vi "AttTGCFix.vi"(0 "slope (m)":dbl[][](array[numeric]) format="%.2f", 1 "Corrections":T1(ring), 5 "intercept (b) out":dbl[][](array[numeric]) format="%.2f", 7 "midband fit in":dbl[][](array[numeric]) format="%.2f", 9 "midband correction":dbl[](array[numeric]) format="%.2f", 11 "slope correction":dbl[](array[numeric]) format="%.2f", 13 "Fit band":T2 {"center freq" format="%.2f"; "stop freq" format="%.2f"; "start" format="%.2f"}) -> (4 "slope":dbl[][](array[numeric]) format="%.2f", 6 "intercept":dbl[][](array[numeric]) format="%.2f", 8 "midband fit":dbl[][](array[numeric]) format="%.2f")   [LabVIEW 2022 SP3]
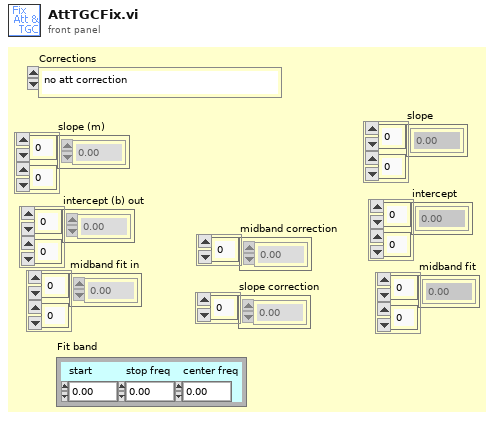
[diagram p1: front panel]
types:
  T1 = enum16{"no att correction", "att correction", "B&K 3535, TGC & att corr"}
  T2 = cluster{"start":dbl, "stop freq":dbl, "center freq":dbl}
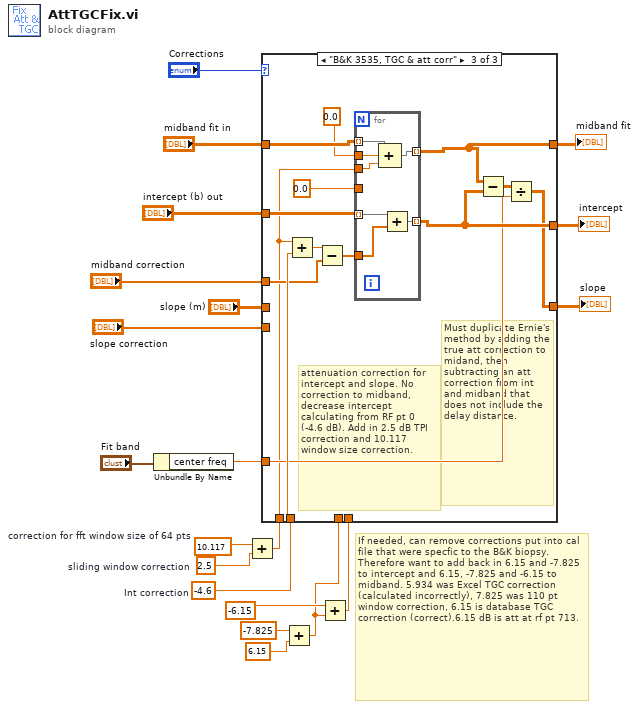
[diagram p0: block diagram]
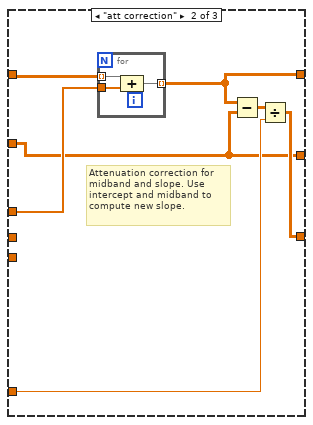
[diagram p3: hidden frame]
diagram:
  w2 = -4.6  # Int correction
  w8 = 10.117  # correction for fft window size of 64 pts
  w9 = 2.5  # sliding window correction
  # "If needed, can remove corrections put into cal file that were specfic to the B&K biopsy. Therefore want to add back in 6.15 and -7.825 to intercept and 6.15, -7.825 and -6.15 to midband. 5.934 was Excel TGC correction (calculated incorrectly), 7.825 was 110 pt window correction, 6.15 is database TGC correction (correct).6.15 dB is att at rf pt 713."
  n1 = Unbundle By Name("Fit band") -> ("center freq"=w3:dbl)
  n2 = Add(x=w8, y=w9) -> (x+y=w7:dbl)
  n3 = Add(x=-7.825, y=6.15) -> (x+y=w6:dbl)
  n4 = Add(x=-6.15, y=w6) -> (x+y=w5:dbl)
  n5 = case shown="\"B&K 3535, TGC & att corr\"" "Corrections" {
    tunnel: "slope correction" -> [_ _ _]
    tunnel: "slope (m)" -> [w22 _ _]
    tunnel: [w22 w28 w40] -> w20
    tunnel: [w23 w26 w41] -> w19
    tunnel: "intercept (b) out" -> [w23 w26 w44]
    tunnel: "midband fit in" -> [w21 w25 w45]
    tunnel: [w21 w24 w42] -> w18
    tunnel: "midband correction" -> [_ w30 w38]
    tunnel: w5 -> [_ _ _]
    tunnel: w6 -> [_ _ _]
    tunnel: w7 -> [_ _ w37]
    tunnel: w3 -> [_ w27 w39]
    tunnel: w2 -> [_ _ w46]
    frame "no att correction", Default {
    }
    frame "att correction" {
      # "Attenuation correction for midband and slope. Use intercept and midband to compute new slope."
      n6 = for {
        tunnel: w25 -> [w33] mode=indexing
        tunnel: w30 -> [w32]
        tunnel: [w31] -> w24 mode=indexing
        n7 = Compound Arithmetic op=ADD(w33, w32) -> (w31:dbl[])
      }
      n8 = Subtract(x=w24, y=w26) -> (x-y=w29:dbl[][])
      n9 = Divide(x=w29, y=w27) -> (x/y=w28:dbl[][])
    }
    frame "B&K 3535, TGC & att corr" {
      # "Must duplicate Ernie's method by adding the true att correction to midand, then subtracting an att correction from int and midband that does not include the delay distance."
      # "attenuation correction for intercept and slope. No correction to midband, decrease intercept calculating from RF pt 0 (-4.6 dB). Add in 2.5 dB TPI correction and 10.117 window size correction."
      n10 = Add(x=w37, y=w46) -> (x+y=w34:dbl)
      n11 = Subtract(x=w34, y=w38) -> (x-y=w47:dbl[])
      n12 = for {
        tunnel: w44 -> [w54] mode=indexing
        tunnel: [w53] -> w41 mode=indexing
        tunnel: w47 -> [w52]
        tunnel: w45 -> [w51] mode=indexing
        tunnel: w37 -> [w48]
        tunnel: [w50] -> w42 mode=indexing
        tunnel: 0.0 -> [w49]
        tunnel: 0.0 -> [_]
        n13 = Compound Arithmetic op=ADD(w51, w49, w48) -> (w50:dbl[])
        n14 = Add(x=w54, y=w52) -> (x+y=w53:dbl[])
      }
      n15 = Subtract(x=w42, y=w41) -> (x-y=w43:dbl[][])
      n16 = Divide(x=w43, y=w39) -> (x/y=w40:dbl[][])
    }
  }
  "slope" <- w20
  "intercept" <- w19
  "midband fit" <- w18
